vi "Read Pulse Recorder Configuration.vi"(8 "error in (no error)":errorcluster, 11 "Lockin Digitizer in":refnum<class "Lockin Digitizer.lvclass">) -> (0 "error out":errorcluster, 2 "Configuration":T1={"Post-trigger delay"=0.01, "Post-trigger duration"=0.1, "Rate"=1000000.0, "Ranges"=[10.0], "Re-name channels"=[], "Active channels"="0:1", "External clock"=FALSE} {"Rate" format="%#_8pHz"; "Post-trigger duration" format="%#_6ps"; "Post-trigger delay" format="%#_6ps"; "Ranges" format="%#_6pV"}, 3 "Lockin Digitizer out":refnum<class "Lockin Digitizer.lvclass">)   [LabVIEW 2021, in "Lockin Digitizer.lvclass"]
uses:
  Lockin Digitizer.lvclass
  NHMFL_Core/Libraries/Instruments/Pulse Driver/Pusle Driver Configuration.ctl
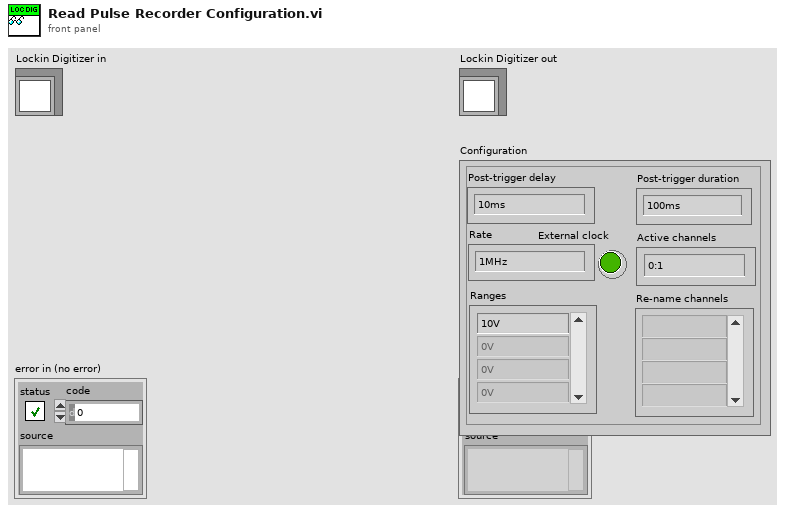
[diagram p1: front panel]
types:
  T1 = typedef "Pusle Driver Configuration.ctl" = cluster{"Post-trigger delay":dbl, "Post-trigger duration":dbl, "Rate":dbl, "Ranges":dbl[], "Re-name channels":string[], "Active channels":string, "External clock":bool}
  T2 = typedef "Lockin Digitizer Configuration.ctl" = cluster{"Post-trigger delay":dbl, "Post-trigger duration":dbl, "Rate":dbl, "Ranges":dbl[], "Re-name channels":string[], "Active channels":string, "External\nclock":bool, "Frequencies":dbl[], "Time\nconstant":dbl, "Output \namplitudes":dbl[], "Lock-in #":i32[], "Input\nchannles":string[]}
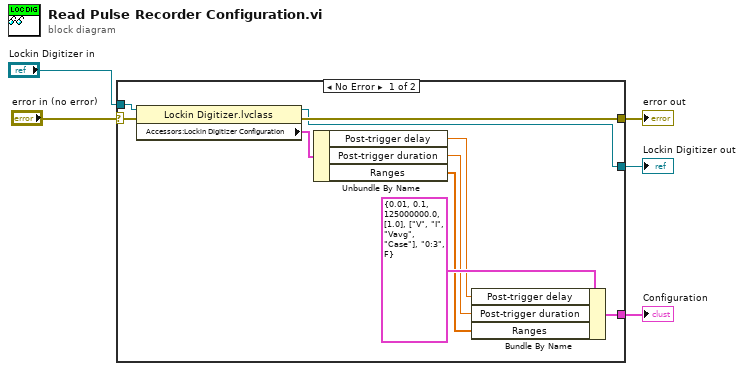
[diagram p0: block diagram]
diagram:
  n1 = case shown="No Error" "error in (no error)" {
    selector: "error in (no error)" -> [w14 w16]
    tunnel: [w13 w16] -> w1
    tunnel: [w12 w17] -> w2
    tunnel: "Lockin Digitizer in" -> [w15 w17]
    tunnel: [w10 _] -> w3
    frame No Error {
      n2 = property class="Lockin Digitizer.lvclass"(reference=w15, error in=w14) -> (reference out=w12:refnum<class "Lockin Digitizer.lvclass">, error out=w13:errorcluster, "Accessors:Lockin Digitizer Configuration"=w6:T2)
      n3 = Unbundle By Name(w6) -> ("Post-trigger delay"=w9:dbl, "Post-trigger duration"=w8:dbl, "Ranges"=w7:dbl[])
      n4 = Bundle By Name(cluster=T1 {"Post-trigger delay"=0.01, "Post-trigger duration"=0.1, "Rate"=125000000.0, "Ranges"=[1.0], "Re-name channels"=["V", "I", "Vavg", "Case"], "Active channels"="0:3", "External clock"=FALSE} ("Configuration"), "Post-trigger delay"=w9, "Post-trigger duration"=w8, "Ranges"=w7) -> (w10:T1)
    }
    frame Error {
    }
  }
  "error out" <- w1
  "Lockin Digitizer out" <- w2
  "Configuration" <- w3
